vi "Help.Load.vi"(8 "error in (no error)":errorcluster, 11 "Web Browser Reference":refnum<k7>(container)) -> (0 "error out":errorcluster)   [LabVIEW 2015]
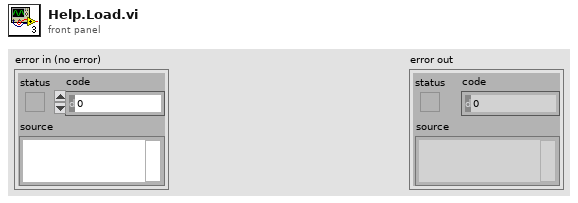
[diagram p1: front panel]
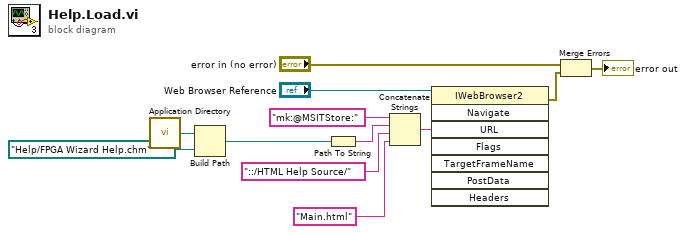
[diagram p0: block diagram]
diagram:
  n1 = call <vilib>:"Application Directory.vi"() -> ("Application Directory"=w1:path)
  n2 = Build Path(base path=w1, name or relative path=path "Help/FPGA Wizard Help.chm" ("stripped path")) -> (appended path=w3:path)
  n3 = Path To String(path=w3) -> (string=w10:string)
  n4 = Concatenate Strings("mk:@MSITStore:" ("string"), w10, "::/HTML Help Source/" ("name or relative path"), "Main.html" ("HTML File")) -> (w4:string)
  n5 = invoke class="IWebBrowser2" method="Navigate"(reference="Web Browser Reference", "URL"=w4) -> (error out=w7:errorcluster)  [unwired: 6 in, 7 out]
  n6 = Merge Errors("error in (no error)", w7) -> (→"error out":errorcluster)
